vi "Write Data.vi"(10 "数据":i32, 11 "Alpha任务消息输入":refnum<class "Alpha任务消息.lvclass">) -> (3 "Alpha任务消息输出":refnum<class "Alpha任务消息.lvclass">)   [LabVIEW 2013, in "Alpha操作者.lvlib" / "Alpha任务消息.lvclass"]
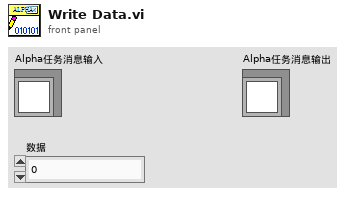
[diagram p1: front panel]
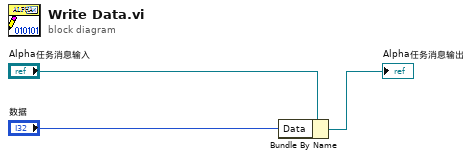
[diagram p0: block diagram]
diagram:
  n1 = Bundle By Name(cluster="Alpha任务消息输入", "Data"="数据") -> (→"Alpha任务消息输出":refnum<class "Alpha任务消息.lvclass">)
